vi "get data definition.vi"(10 "channel classification":T1, 11 "My Awesome Control Modules runtime in":refnum<class "My Awesome Control Modules runtime.lvclass">) -> (1 "valid?":bool, 2 "index cluster":variant, 3 "My Awesome Control Modules runtime out":refnum<class "My Awesome Control Modules runtime.lvclass">)   [LabVIEW 2013, in "My Awesome Control Modules runtime.lvclass"]
uses:
  My Awesome Control Modules runtime.lvclass
  input user data.ctl
  output user data.ctl
  parameter user data.ctl
  result user data.ctl
  <vilib>/NI/Tag Bus Module Framework/channel/channel classification.ctl
  <vilib>/NI/Tag Bus Module Framework/channel/TBM channel.lvclass
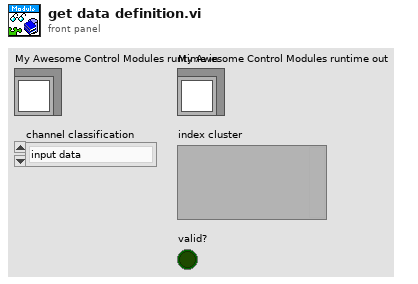
[diagram p1: front panel]
types:
  T1 = typedef "TBM channel.lvclass/channel classification.ctl" = enum16{"input data", "output data", "processing parameter", "processing result"}
  T2 = typedef "My Awesome Control Modules runtime.lvclass/input user data.ctl" = cluster{"asd":dbl}
  T3 = typedef "My Awesome Control Modules runtime.lvclass/output user data.ctl" = cluster{"fmwk_placeholder":i32}
  T4 = typedef "My Awesome Control Modules runtime.lvclass/parameter user data.ctl" = cluster{"Temperature":dbl, "setpoint":dbl, "output range high":dbl, "output range low":dbl, "Kc":dbl, "Ti":dbl, "Td":dbl, "Fan on?":bool}
  T5 = typedef "My Awesome Control Modules runtime.lvclass/result user data.ctl" = cluster{"fan":dbl, "lamp":dbl}
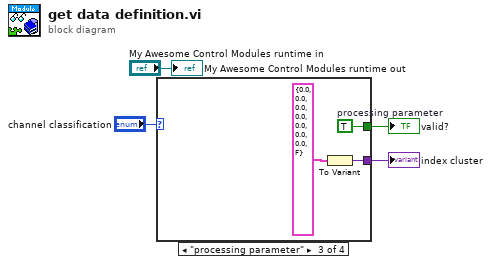
[diagram p0: block diagram]
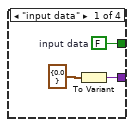
[diagram p2: hidden frame]
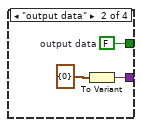
[diagram p3: hidden frame]
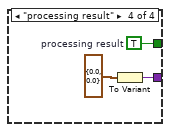
[diagram p4: hidden frame]
diagram:
  n1 = case shown="\"processing parameter\"" "channel classification" {
    tunnel: [w6 w10 w13 w16] -> w2
    tunnel: [w5 w9 w12 w15] -> w1
    frame "input data" {
      w5 = FALSE  # input data
      n2 = To Variant(anything=T2 {"asd"=0.0} ("Inputs from system")) -> (Variant=w6:variant)
    }
    frame "output data" {
      w9 = FALSE  # output data
      n3 = To Variant(anything=T3 {"fmwk_placeholder"=0} ("Outputs to system")) -> (Variant=w10:variant)
    }
    frame "processing parameter" {
      w12 = TRUE  # processing parameter
      n4 = To Variant(anything=T4 {"Temperature"=0.0, "setpoint"=0.0, "output range high"=0.0, "output range low"=0.0, "Kc"=0.0, "Ti"=0.0, "Td"=0.0, "Fan on?"=FALSE} ("Parameters to process")) -> (Variant=w13:variant)
    }
    frame "processing result" {
      w15 = TRUE  # processing result
      n5 = To Variant(anything=T5 {"fan"=0.0, "lamp"=0.0} ("Results from processing")) -> (Variant=w16:variant)
    }
  }
  "index cluster" <- w2
  "valid?" <- w1
  "My Awesome Control Modules runtime out" <- "My Awesome Control Modules runtime in"
